vi "Unregister.vi"(8 "error in":errorcluster, 11 "Read Event in":refnum<class "Read Event.lvclass">) -> (0 "error out":errorcluster, 3 "Read Event out":refnum<class "Read Event.lvclass">)   [LabVIEW 2018, in "PCANBasic.lvlib" / "Read Event.lvclass"]
uses:
  Read Event.lvclass
  Message Waiter/Message Waiter.lvclass
  Read Event.lvclass/Read Event.ctl
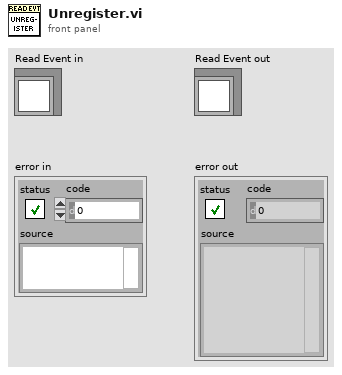
[diagram p1: front panel]
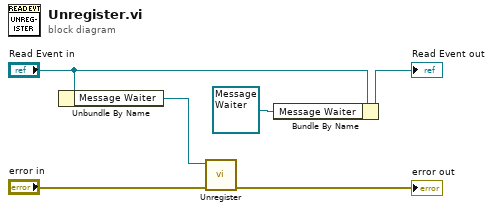
[diagram p0: block diagram]
diagram:
  n1 = Unbundle By Name("Read Event in") -> ("Message Waiter"=w6:refnum<class "Message Waiter.lvclass">)
  n2 = call-dynamic "Unregister.vi"("error in"="error in", "Message Waiter in"=w6) -> ("error out"=→"error out":errorcluster)  [unwired: 8 in, 1 out]
  n3 = Bundle By Name(cluster="Read Event in", "Message Waiter"=refnum<class "Message Waiter.lvclass"> refnum ("IWait for Message")) -> (→"Read Event out":refnum<class "Read Event.lvclass">)
